vi "Get Formatter.vi"(8 "error in":errorcluster, 11 "FileHandler":refnum<class "NetworkHandler.lvclass">) -> (0 "error out":errorcluster, 2 "Formatter":refnum<class "Formatter.lvclass">, 3 "FileHandler out":refnum<class "NetworkHandler.lvclass">)   [LabVIEW 2024]
doc: "Returns the Formatter for this handler.\n\n____\nHAMPEL SOFTWARE ENGINEERING v2.2.2 (2025-01-16 15:41)"
uses:
  <vilib>/Hampel Software Engineering/HSE Logger/Formatter/Formatter.lvclass
  NetworkHandler.lvclass
  NetworkHandler.lvclass/NetworkHandler.ctl
  C:/Program Files (x86)/National Instruments/LabVIEW 2024/vi.lib/Hampel Software Engineering/HSE Logger/Handler/Handler.lvclass
  C:/DevOps/CORTEX/X_T2126_SDE_Rig_CAT/HSEExtensions/NetworkHandler/NetworkHandler.lvclass
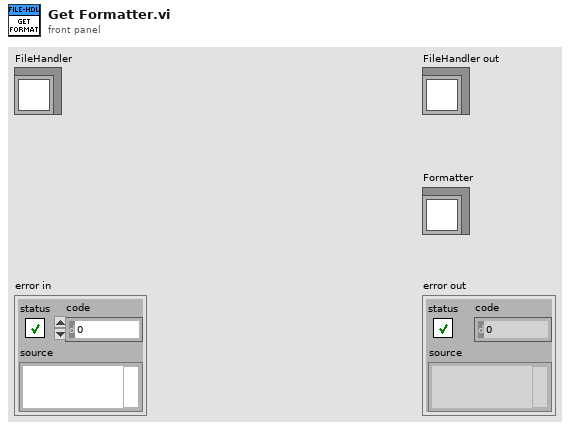
[diagram p1: front panel]
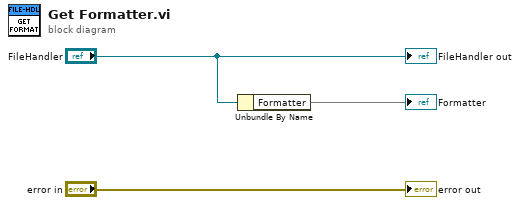
[diagram p0: block diagram]
diagram:
  n1 = Unbundle By Name("FileHandler") -> ("Formatter"=→"Formatter")
  "error out" <- "error in"
  "FileHandler out" <- "FileHandler"
